vi "Module Identities.vi"(8 "error in (no error)":errorcluster, 11 "Historian Module in":refnum<class "Historian Module.lvclass">) -> (0 "error out":errorcluster, 2 "Identities":refnum<class "Identity.lvclass">[](array[class]), 3 "Historian Module out":refnum<class "Historian Module.lvclass">)   [LabVIEW 2020, in "VolatusHistorian.lvlib" / "Historian Module.lvclass"]
uses:
  Historian Module.lvclass
  Volatus/Identity/Identity.lvclass
  Historian Module.lvclass/Historian Module.ctl
  Historian Identity/Historian Identity.lvclass
  C:/dev/lv20CE/relink/lv-volatus/VolatusHistorian/Historian Identity/Historian Identity.lvclass
  C:/dev/lv20CE/relink/lv-volatus/Volatus/Identity/Identity.lvclass
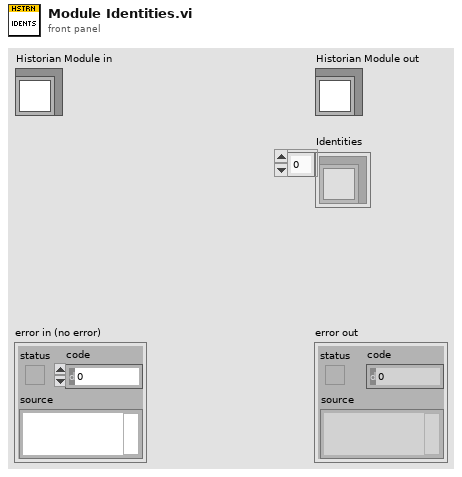
[diagram p1: front panel]
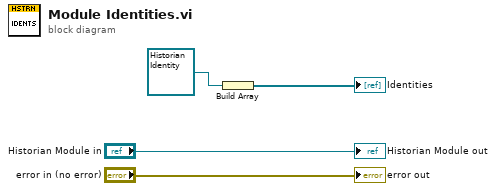
[diagram p0: block diagram]
diagram:
  n1 = Build Array(refnum<class "Historian Identity.lvclass"> refnum ("VolatusHistorian.lvlib:Historian Identity.lvclass")) -> (→"Identities":refnum<class "Historian Identity.lvclass">[])
  "error out" <- "error in (no error)"
  "Historian Module out" <- "Historian Module in"
